vi "SetMotorSpeeds.vi"(0 "Right Motor PWM":dbl(slide) scale=-1.0..1.0, 1 "Left Motor PWM":dbl(slide) scale=-1.0..1.0) -> ()   [LabVIEW 2015, in "Overlord2017.lvlib"]
uses:
  Overlord2017.lvlib
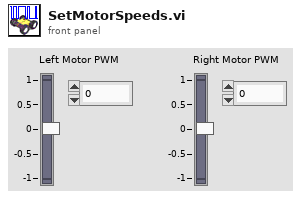
[diagram p1: front panel]
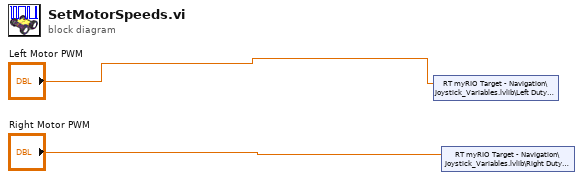
[diagram p0: block diagram]
diagram:
  n1 = shared-variable "RT myRIO Target - Navigation\\Joystick_Variables.lvlib\\Left Duty Cycle"("Left Motor PWM") -> ()  [unwired: 1 in, 1 out]
  n2 = shared-variable "RT myRIO Target - Navigation\\Joystick_Variables.lvlib\\Right Duty Cycle"("Right Motor PWM") -> ()  [unwired: 1 in, 1 out]
